vi "Brightcoveload.vi"() -> ()   [LabVIEW 2026]
uses:
  <vilib>/sklein/WebView2/Webview2 Lib/WebView2 Control Object/Paths.ctl
  <vilib>/sklein/WebView2/Webview2 Lib/WebView2 Control Object/Core Env Options.ctl
  <vilib>/sklein/WebView2 QControl/WebView2 QControl/WebView2 QControl/WebView2 QControl.lvclass/WebView2 QControl.ctl
  <userlib>/_lava_lib_tree_control.llb/CommunityTreeAPITYPEDEF - DataStore Command.ctl
  9dcc2fe5-36b0-449a-ab0d-001457c950c8.vi
  5299e24a-5130-419c-9a3c-199b24d92175.vi
  <vilib>/sklein/WebView2 QControl/WebView2 QControl/WebView2 QControl/Write Document Source.vi
  <vilib>/sklein/WebView2 QControl/WebView2 QControl/WebView2 QControl/Read Events.vi
  <vilib>/sklein/WebView2/Webview2 Lib/WebView2 Control Object/Read Events.vi
  <vilib>/sklein/WebView2/Webview2 Lib/WebView2 Control Object/Write Document Source.vi
  <vilib>/sklein/WebView2/Webview2 Lib/WebView2 Control Object/Register Events.vi
  <vilib>/JDP Science/JSONtext/Variant to JSON Text.vi
  <vilib>/JDP Science/JSONtext/LVClass Serializer/JSONtext LVClass Serializer.lvclass
  <vilib>/sklein/WebView2 QControl/WebView2 QControl/WebView2 QControl/WebView2 QControl.lvclass
  <vilib>/sklein/WebView2/Webview2 Lib/WebView2 Control Object/WebView2 Control.lvclass
  <vilib>/sklein/WebView2/Libs/Microsoft.Web.WebView2.WinForms.dll
panel:
  out "<JSON>":string
  in  "WebView2":refnum<k24>(container)
  in  "Tree":string(tree)
  in  "Tree 2":string(tree)
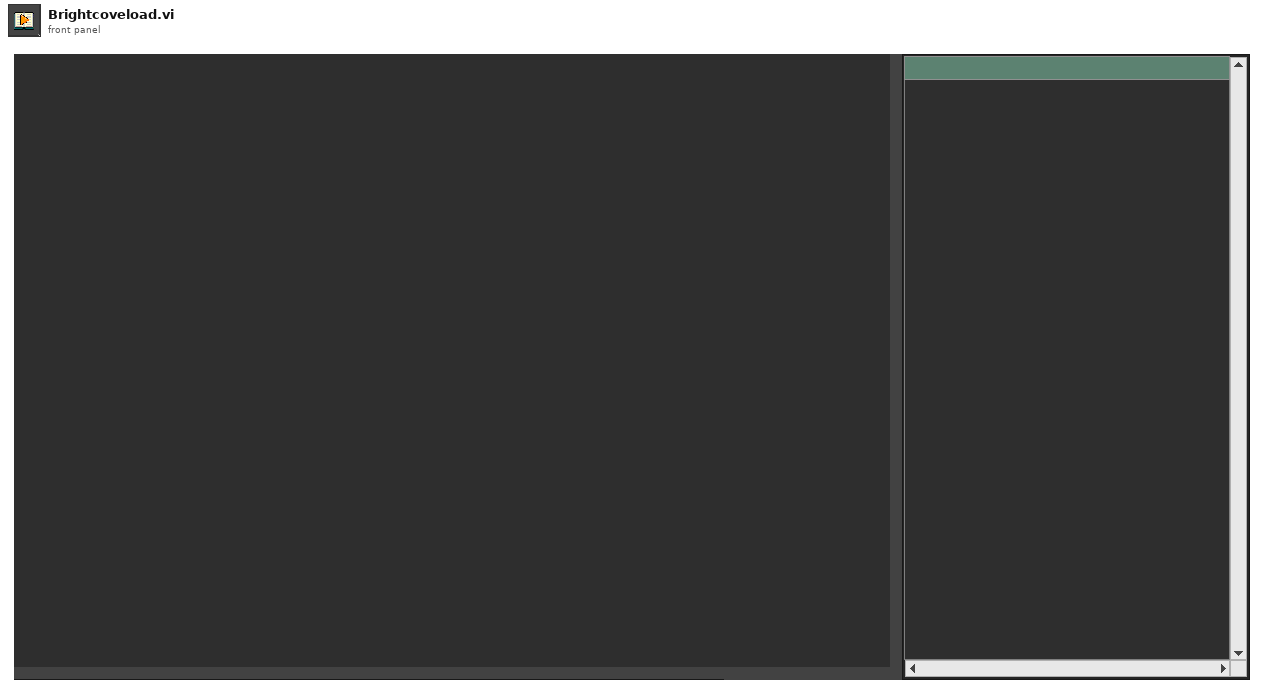
[diagram p1: front panel]
types:
  T1 = typedef "WebView2.lvlib/WebView2 Control.lvclass/Core Env Options.ctl" = cluster{"additionalBrowserArguments":string, "language":string, "targetCompatibleBrowserVersion":string, "allowSingleSignOnUsingOSPrimaryAccount":bool}
  T2 = typedef "WebView2.lvlib/WebView2 Control.lvclass/Paths.ctl" = cluster{"Webview2 Native":path, "Edge Application":path, "User Data":path}
  T3 = typedef "WebView2.lvlib/WebView2 Control.lvclass/Events.ctl" = cluster{"Navigation Complete Event":refnum<user-event>, "Source Changed Event":refnum<user-event>, "Document Title Changed Event":refnum<user-event>, "Status Bar Text Changed":refnum<user-event>, "Web Message Received":refnum<user-event>, "Window Close Requested":refnum<user-event>, "DOM Loaded":refnum<user-event>, "Navigation Started Event":refnum<user-event>}
  T4 = typedef "imagedata.ctl" = cluster{"image type":i32, "image depth":i32, "image":u8[], "mask":u8[], "colors":u32[], "Rectangle":cluster{"left":i16, "top":i16, "right":i16, "bottom":i16}}
  T5 = typedef "CommunityTreeAPITYPEDEF - DataStore Command.ctl" = enum16{"Init", "Add", "Get", "Clear Tree", "Clear All", "Modify"}
  T6 = typedef "LVRectTypeDef.ctl" = cluster{"Left":i16, "Top":i16, "Right":i16, "Bottom":i16}
  T7 = enum16{"No Scaling", "Scale All Objects", "Scale Single Object"}
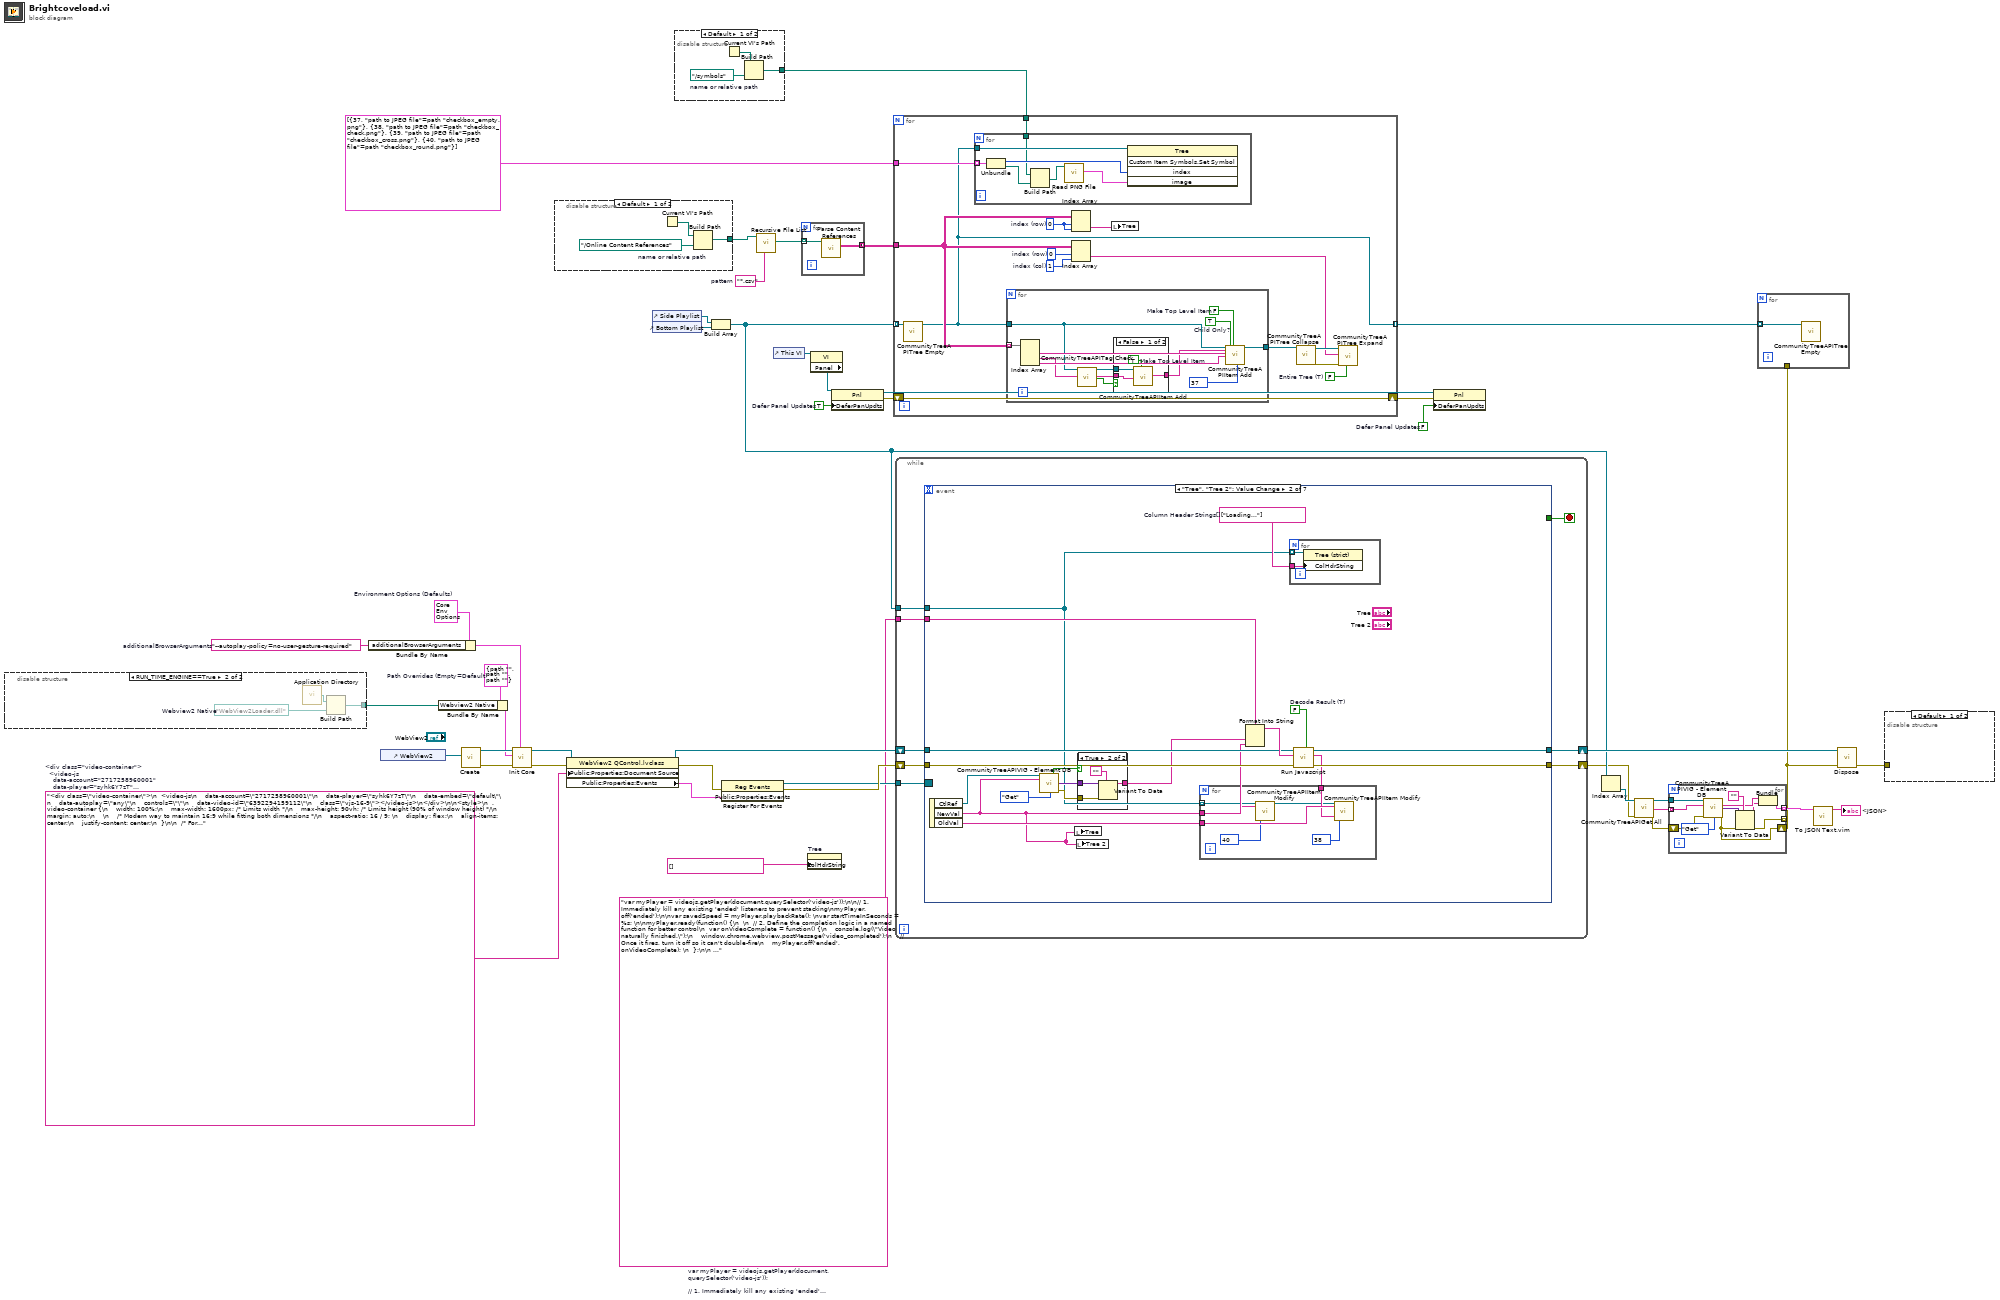
[diagram p0: block diagram]
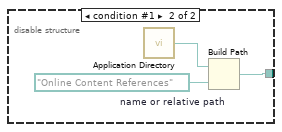
[diagram p2: hidden frame]
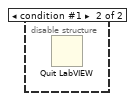
[diagram p4: hidden frame]
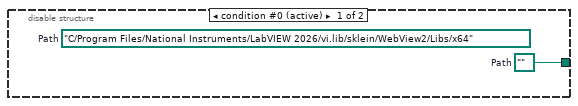
[diagram p5: hidden frame]
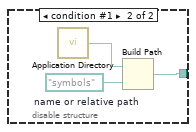
[diagram p6: hidden frame]
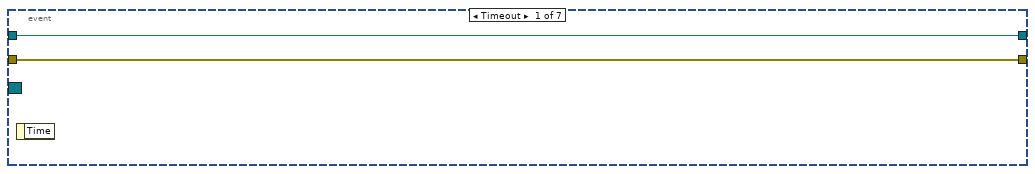
[diagram p7: hidden frame]
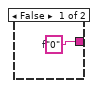
[diagram p8: hidden frame]
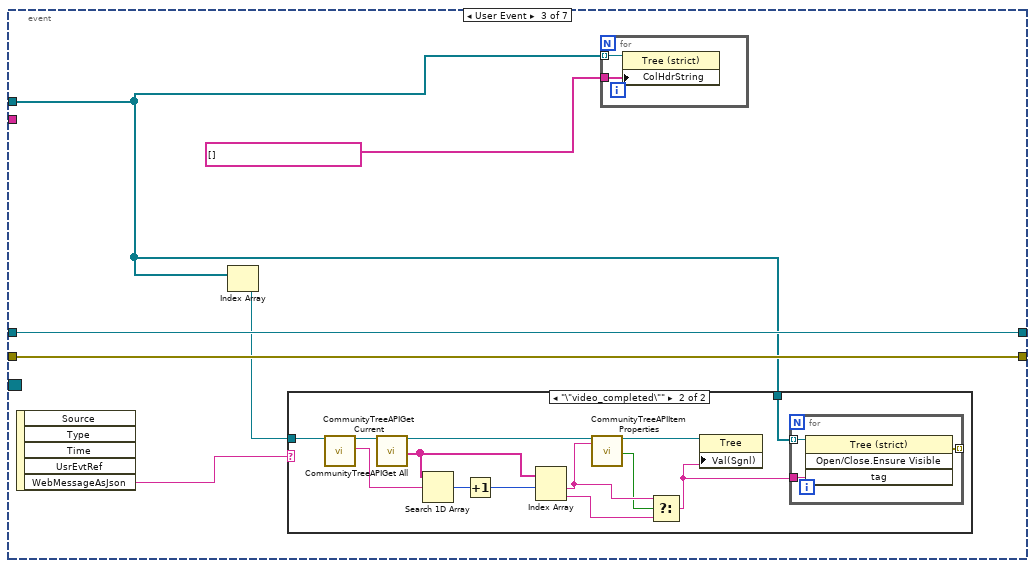
[diagram p9: hidden frame]
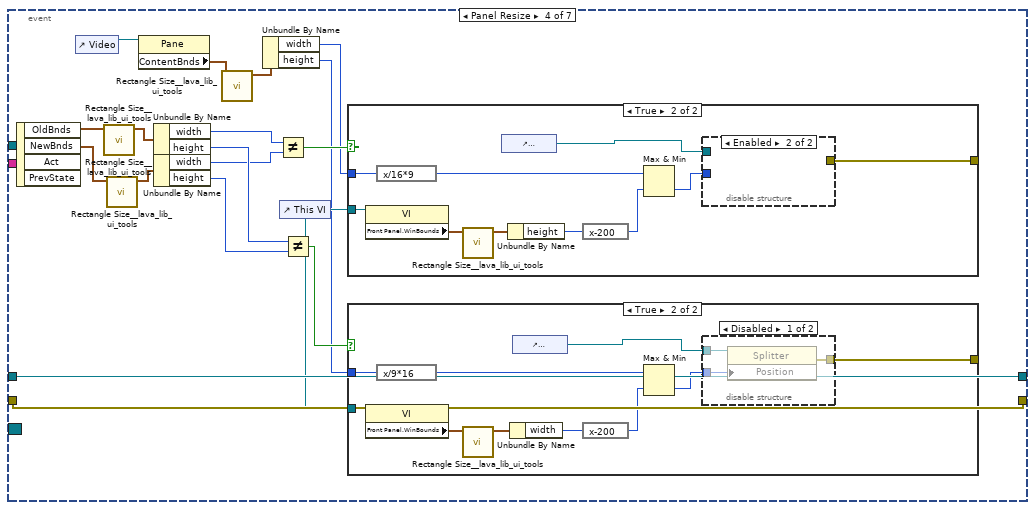
[diagram p11: hidden frame]
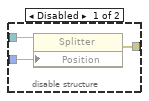
[diagram p15: hidden frame]
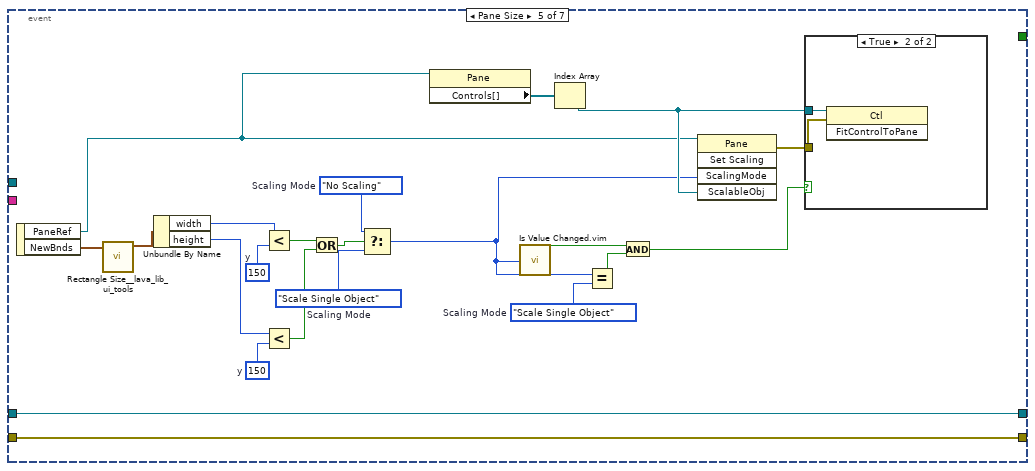
[diagram p16: hidden frame]
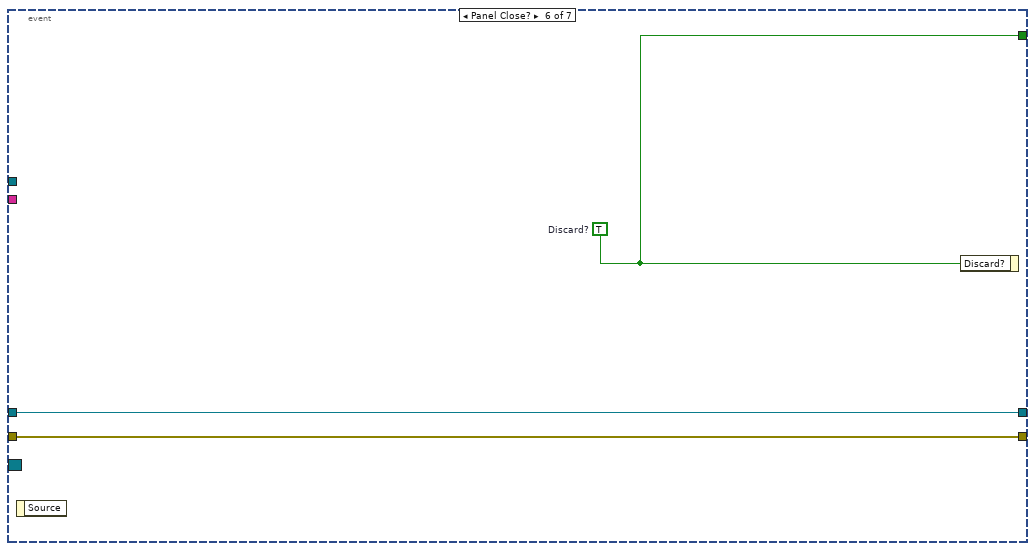
[diagram p18: hidden frame]
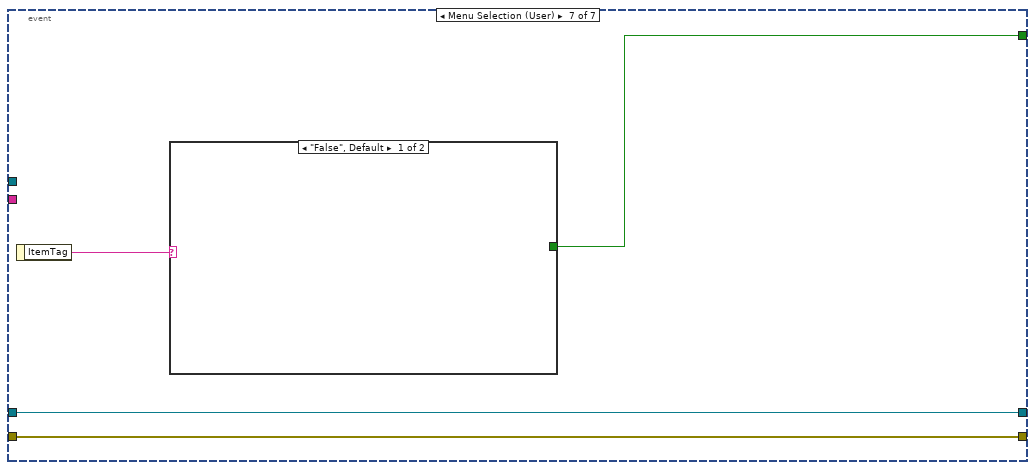
[diagram p19: hidden frame]
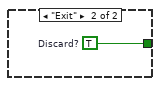
[diagram p20: hidden frame]
diagram:
  w2 = "--autoplay-policy=no-user-gesture-required"  # additionalBrowserArguments
  w4 = T1 {"additionalBrowserArguments"="--autoplay-policy=no-user-gesture-required", "language"="", "targetCompatibleBrowserVersion"="", "allowSingleSignOnUsingOSPrimaryAccount"=FALSE}  # Environment Options (Defaults)
  w16 = "*.csv"  # pattern
  w22 = FALSE  # Defer Panel Updates
  w25 = TRUE  # Defer Panel Updates
  w14 = "var myPlayer = videojs.getPlayer(document.querySelector('video-js'));\n\n// 1. Immediately kill any existing 'ended' listeners to prevent stacking\nmyPlayer.off('ended');\n\nvar savedSpeed = myPlayer.playbackRate(); \nvar startTimeInSeconds = %s; \n\nmyPlayer.ready(function() {\n  \n  // 2. Define the completion logic in a named function for better control\n  var onVideoComplete = function() {\n    console.log(\"Video naturally finished.\");\n    window.chrome.webview.postMessage('video_completed');\n    // Once it fires, turn it off so it can't double-fire\n    myPlayer.off('ended', onVideoComplete); \n  };\n\n  myPlayer.catalog.getVideo('%s', function(error, video) {\n    if (!error) {\n      // 3. Pause and reset the current source before loading the new one\n      myPlayer.pause();\n      \n      myPlayer.catalog.load(video);\n      \n      myPlayer.one('loadedmetadata', function() {\n        myPlayer.playbackRate(savedSpeed);  \n        myPlayer.currentTime(startTimeInSeconds); \n        \n        // 4. Only attach the 'ended' listener AFTER the new video is ready\n        myPlayer.on('ended', onVideoComplete);\n\n        myPlayer.play(); \n        window.chrome.webview.postMessage('abc'); \n      });\n    }\n  });\n});\nmyPlayer.currentTime();"  # var myPlayer = videojs.getPlayer(document.querySelector('video-js'));  // 1. Immediately kill any existing 'ended' listeners to prevent stacking myPlayer.off('ended');  var savedSpeed = myPlayer.playbackRate();  var startTimeInSeconds = %s;   myPlayer.ready(function() {      // 2. Define the completion logic in a named function for better control   var onVideoComplete = function() {     console.log("Video naturally finished.");     window.chrome.webview.postMessage('video_completed');     // Once it fires, turn it off so it can't double-fire     myPlayer.off('ended', onVideoComplete);    };    myPlayer.catalog.getVideo('%s', function(error, video) {     if (!error) {       // 3. Pause and reset the current source before loading the new one       myPlayer.pause();              myPlayer.catalog.load(video);              myPlayer.one('loadedmetadata', function() {         myPlayer.playbackRate(savedSpeed);           myPlayer.currentTime(startTimeInSeconds);                   // 4. Only attach the 'ended' listener AFTER the new video is ready         myPlayer.on('ended', onVideoComplete);          myPlayer.play();          window.chrome.webview.postMessage('abc');        });     }   }); }); myPlayer.currentTime();
  w34 = T2 {"Webview2 Native"=path "", "Edge Application"=path "", "User Data"=path ""}  # Path Overrides (Empty=Default)
  w40 = "<div class=\"video-container\">\n  <video-js\n    data-account=\"2717258960001\"\n    data-player=\"syhk6Y7zT\"\n    data-embed=\"default\"\n    data-autoplay=\"any\"\n    controls=\"\"\n    data-video-id=\"6392294159112\"\n    class=\"vjs-16-9\"></video-js>\n</div>\n\n<style>\n  .video-container {\n    width: 100%;\n    max-width: 1600px; /* Limits width */\n    max-height: 90vh; /* Limits height (90% of window height) */\n    margin: auto;\n    \n    /* Modern way to maintain 16:9 while fitting both dimensions */\n    aspect-ratio: 16 / 9; \n    display: flex;\n    align-items: center;\n    justify-content: center;\n  }\n\n  /* Force the video-js element to fill this constrained container */\n  .video-container video-js {\n    width: 100% !important;\n    height: 100% !important;\n    position: relative !important;\n    padding-top: 0 !important; /* Overrides the default vjs-16-9 padding */\n  }\n</style>\n<script\n  src=\"https://players.brightcove.net/2717258960001/syhk6Y7zT_default/index.min.js\">\n</script>\n"  # <div class="video-container">   <video-js     data-account="2717258960001"     data-player="syhk6Y7zT"     data-embed="default"     data-autoplay="any"     controls=""     data-video-id="6392294159112"     class="vjs-16-9"></video-js> </div>  <style>   .video-container {     width: 100%;     max-width: 1600px; /* Limits width */     max-height: 90vh; /* Limits height (90% of window height) */     margin: auto;          /* Modern way to maintain 16:9 while fitting both dimensions */     aspect-ratio: 16 / 9;      display: flex;     align-items: center;     justify-content: center;   }    /* Force the video-js element to fill this constrained container */   .video-container video-js {     width: 100% !important;     height: 100% !important;     position: relative !important;     padding-top: 0 !important; /* Overrides the default vjs-16-9 padding */   } </style> <script   src="https://players.brightcove.net/2717258960001/syhk6Y7zT_default/index.min.js"> </script>
  n1 = disable-structure shown="RUN_TIME_ENGINE==True" {
    disable-tunnel: [w47 w48] -> w27
    frame condition #0 (active) {
      (unwired) path "C:/Program Files/National Instruments/LabVIEW 2026/vi.lib/sklein/WebView2/Libs/x64"  # Path
      w47 = path ""  # Path
    }
    frame condition #1 {
      w49 = path "WebView2Loader.dll"  # Webview2 Native
      n2 = call <vilib>:"Application Directory.vi"() -> ("Application Directory"=w50:path)
      n3 = Build Path(base path=w50, name or relative path=w49) -> (appended path=w48:path)
    }
  }
  n4 = Bundle By Name(cluster=w4, "additionalBrowserArguments"=w2) -> (w3:T1)
  n5 = control-ref of="WebView2"() -> (w44:refnum<vi>)
  n6 = Bundle By Name(cluster=w34, "Webview2 Native"=w27) -> (w32:T2)
  n7 = call <vilib>:"Create.vi"("WebView2 Control Ref"=w44) -> ("error out"=w38:errorcluster, "WebView2 Control out"=w43:refnum<class "WebView2 QControl.lvclass">)  [unwired: 9 in]
  n8 = call <vilib>:"Init Core.vi"("Environment Options (Defaults)"=w3, "error in (no error)"=w38, "Path Overrides (Empty=Default)"=w32, "WebView2 Control in"=w43) -> ("error out"=w42:errorcluster, "WebView2 Control out"=w37:refnum<class "WebView2 QControl.lvclass">)  [unwired: 6 in]
  n9 = disable-structure shown="Default" {
    disable-tunnel: [w51 w54] -> w17
    frame condition #0 (active) {
      w53 = path "../Online Content References"  # name or relative path
      n10 = Current VI's Path() -> (path=w52:path)
      n11 = Build Path(base path=w52, name or relative path=w53) -> (appended path=w51:path)
    }
    frame condition #1 {
      w56 = path "Online Content References"  # name or relative path
      n12 = call <vilib>:"Application Directory.vi"() -> ("Application Directory"=w55:path)
      n13 = Build Path(base path=w55, name or relative path=w56) -> (appended path=w54:path)
    }
  }
  n14 = property class="WebView2 QControl.lvclass"(reference=w37, error in=w42, "Public:Properties:Document Source"=w40) -> (reference out=w36:refnum<class "WebView2 QControl.lvclass">, error out=w1:errorcluster, "Public:Properties:Events"=w30:T3)
  n15 = control-ref of="Side Playlist"() -> (w26:refnum<vi>)
  n16 = control-ref of="Bottom Playlist"() -> (w45:refnum<vi>)
  n17 = disable-structure shown="Default" {
    disable-tunnel: [w57 w60] -> w35
    frame condition #0 (active) {
      w59 = path "../symbols"  # name or relative path
      n18 = Current VI's Path() -> (path=w58:path)
      n19 = Build Path(base path=w58, name or relative path=w59) -> (appended path=w57:path)
    }
    frame condition #1 {
      w62 = path "symbols"  # name or relative path
      n20 = call <vilib>:"Application Directory.vi"() -> ("Application Directory"=w61:path)
      n21 = Build Path(base path=w61, name or relative path=w62) -> (appended path=w60:path)
    }
  }
  n22 = Build Array(w26, w45) -> (w13:refnum<vi>[])
  n23 = register-events(error in=w1, w30) -> (reference out=w29:refnum<event-registration>, error out=w46:errorcluster)  [unwired: 1 in]
  n24 = call <vilib>:"Recursive File List.vi"("pattern"=w16, "Folder Path"=w17) -> ("All Files in Dir"=w15:path[])  [unwired: 5 in, 4 out]
  n25 = control-ref of="This VI"() -> (w20:refnum<vi>)
  n26 = for {
    tunnel: [w64] -> w28 mode=concatenating
    tunnel: w15 -> [w63] mode=indexing
    n27 = call "Parse Content References.vi"("file path in"=w63) -> ("transposed array"=w64:string[][])  [unwired: 14 in]
  }
  n28 = property on="Tree" class="Tree (strict)"("ColHdrString"=string[] []) -> ()  [unwired: 2 in, 2 out]
  n29 = property class="VI"(reference=w20) -> ("Panel"=w19:refnum<vi>)  [unwired: 1 in, 2 out]
  n30 = property class="Pnl"(reference=w19, "DeferPanUpdts"=w25) -> (reference out=w21:refnum<vi>, error out=w24:errorcluster)  [unwired: 1 in]
  n31 = for {
    tunnel: w13 -> [w79] mode=indexing
    tunnel: cluster{i32, "path to JPEG file":path}[] [{37, "path to JPEG file"=path "checkbox_empty.png"}, {38, "path to JPEG file"=path "checkbox_check.png"}, {39, "path to JPEG file"=path "checkbox_cross.png"}, {40, "path to JPEG file"=path "checkbox_round.png"}] -> [w78]
    tunnel: w35 -> [w75]
    tunnel: w28 -> [w67]
    shift-right: [w66] -> w23
    shift-left: w24 -> [w66]
    tunnel: [w65] -> w18 mode=indexing
    w69 = 1  # index (col)
    w70 = 0  # index (row)
    w71 = FALSE  # Entire Tree (T)
    w77 = 0  # index (row)
    n32 = call <userlib>:"CommunityTreeAPITree Empty.vi"("Tree Reference In"=w79) -> ("Tree Reference Out"=w65:refnum<vi>)  [unwired: 16 in, 2 out]
    n33 = for {
      tunnel: w65 -> [w86]
      tunnel: w78 -> [w84] mode=indexing
      tunnel: w75 -> [w80]
      n34 = Unbundle(w84) -> (w83:i32, "path to JPEG file"=w82:path)
      n35 = Build Path(base path=w80, name or relative path=w82) -> (appended path=w81:path)
      n36 = call <vilib>:"Read PNG File.vi"("path to PNG file"=w81) -> ("image data"=w85:T4)  [unwired: 8 in, 2 out]
      n37 = invoke class="Tree" method="Custom Item Symbols.Set Symbol"(reference=w86, "index"=w83, "image"=w85) -> ()  [unwired: 2 in, 5 out]
    }
    n38 = for {
      tunnel: w67 -> [w99] mode=indexing
      tunnel: w65 -> [w94]
      tunnel: [w87] -> w74
      w88 = TRUE  # Child Only?
      w96 = FALSE  # Make Top Level Item
      n39 = Index Array(array=w99) -> (element #1=w97:string, element #2=w93:string, element #3=w98:string)  [unwired: 3 in]
      n40 = call <userlib>:"CommunityTreeAPITag Check.vi"("Tree Reference In"=w94, "Input Tag"=w93) -> ("Tree Reference Out"=w92:refnum<vi>, "Duplicate Tag"=w91:string, "Tag OK"=w89:bool)  [unwired: 14 in, 1 out]
      n41 = case shown="False" w89 {
        tunnel: w92 -> [w103 _]
        tunnel: w91 -> [w102 w104]
        tunnel: [w100 w104] -> w90
        frame False {
          w101 = TRUE  # Make Top Level Item
          n42 = call <userlib>:"CommunityTreeAPIItem Add.vi"("Tree Reference In"=w103, "New Text Value"=w102, "Make Top Level Item"=w101) -> ("Created Tag"=w100:string)  [unwired: 14 in, 2 out]
        }
        frame True {
        }
      }
      n43 = call <userlib>:"CommunityTreeAPIItem Add.vi"("Tree Reference In"=w94, "Parent Tag (Current)"=w90, "New Tag Value (Same as Text)"=w97, "New Text Value"=w98, "Child Only?"=w88, "Make Top Level Item"=w96, "Symbol Index (0)"=37) -> ("Tree Reference Out"=w87:refnum<vi>)  [unwired: 10 in, 2 out]
    }
    n44 = Index Array(array=w67, index (row)=w77, index (col)=w77) -> (element=w76:string)
    n45 = Index Array(array=w67, index (row)=w70, index (col)=w69) -> (element=w68:string)
    n46 = local write "Tree"(w76) -> ()
    n47 = call <userlib>:"CommunityTreeAPITree Collapse.vi"("Tree Reference In"=w74) -> ("Tree Reference Out"=w73:refnum<vi>, "error out"=w72:errorcluster)  [unwired: 17 in]
    n48 = call <userlib>:"CommunityTreeAPITree Expand.vi"("Tree Reference In"=w73, "Tag To Expand"=w68, "error in (no error)"=w72, "Entire Tree (T)"=w71) -> ()  [unwired: 14 in, 2 out]
  }
  n49 = while {
    shift-right: [w109] -> w6
    shift-left: w46 -> [w112]
    shift-right: [w110] -> w41
    shift-left: w36 -> [w111]
    tunnel: w29 -> [w107]
    tunnel: w14 -> [w106]
    tunnel: w13 -> [w105]
    stop <- w108 stop-if-true
    n50 = event shown="[1] \"Tree\", \"Tree 2\": Value Change" {
      selector: w107 -> [_ _ _ _ _ _ _]
      dyn-events: _ -> [_ _ _ _ _ _ _]
      timeout: _ -> [_ _ _ _ _ _ _]
      tunnel: w112 -> [w113 w130 w151 w187 w235 w240 w244]
      tunnel: w111 -> [w114 w128 w152 w188 w236 w241 w245]
      tunnel: [w114 w132 w152 w188 w236 w241 w245] -> w110
      tunnel: [w113 w131 w151 w187 w235 w240 w244] -> w109
      tunnel: [_ _ _ _ _ w239 w242] -> w108
      tunnel: w106 -> [_ w116 _ _ _ _ _]
      tunnel: w105 -> [_ w115 w147 _ _ _ _]
      event Timeout {
        n51 = event-data() -> ()  [unwired: 1 in, 1 out]
      }
      event "Tree", "Tree 2": Value Change {
        w118 = string[] ["Loading..."]  # Column Header Strings[]
        w127 = FALSE  # Decode Result (T)
        n52 = event-data() -> ("CtlRef"=w122:refnum<vi>, "NewVal"=w117:string, "OldVal"=w126:string)  [unwired: 1 in]
        n53 = call <userlib>:"CommunityTreeAPIVIG - Element DB.vi"("Tree Ref In"=w122, "Element Tag"=w117, "Command"=CommunityTreeAPITYPEDEF_-_DataStore_Command."Get") -> ("Found"=w120:bool, "Tree Element Data Out"=w123:variant, "error out"=w121:errorcluster)  [unwired: 7 in, 3 out]
        n54 = local write "Tree"(w117) -> ()
        n55 = local write "Tree 2"(w117) -> ()
        n56 = case shown="True" w120 {
          tunnel: w123 -> [_ w146]
          tunnel: [w142 w144] -> w119
          tunnel: w121 -> [_ w143]
          frame False {
            w142 = "0"  # f
          }
          frame True {
            n57 = Variant To Data(error in=w143, type="", Variant=w146) -> (data=w144:string)  [unwired: 1 out]
          }
        }
        n58 = Format Into String(format string=w116, w119, w117) -> (resulting string=w129:string)  [unwired: 2 in, 1 out]
        n59 = for {
          tunnel: w118 -> [w134]
          tunnel: w115 -> [w133] mode=indexing
          n60 = property on="Property Node" class="Tree (strict)"(reference=w133, "ColHdrString"=w134) -> ()  [unwired: 1 in, 2 out]
        }
        n61 = call <vilib>:"Run Javascript.vi"("Decode Result (T)"=w127, "error in (no error)"=w130, "javaScript"=w129, "WebView2 Control in"=w128) -> ("error out"=w131:errorcluster, "Result"=w125:string, "WebView2 Control out"=w132:refnum<class "WebView2 QControl.lvclass">)  [unwired: 5 in]
        n62 = for {
          tunnel: w126 -> [w141]
          tunnel: w125 -> [w140]
          tunnel: w115 -> [w139] mode=indexing
          tunnel: w117 -> [w135]
          n63 = call <userlib>:"CommunityTreeAPIItem Modify.vi"("Tree Reference In"=w139, "Tag to Modify (Current)"=w135, "Symbol(-1:No Change)"=40) -> ("Tree Reference Out"=w137:refnum<vi>)  [unwired: 14 in, 2 out]
          n64 = call <userlib>:"CommunityTreeAPIItem Modify.vi"("Tree Reference In"=w137, "Tag to Modify (Current)"=w141, "Element Data"=w140, "Symbol(-1:No Change)"=38) -> ()  [unwired: 13 in, 3 out]
        }
      }
      event User Event {
        n65 = event-data() -> ("WebMessageAsJson"=w149:string)  [unwired: 1 in, 4 out]
        n66 = Index Array(array=w147) -> (element=w148:refnum<vi>)  [unwired: 1 in]
        n67 = case shown="\"\\\"video_completed\\\"\"" w149 {
          tunnel: w148 -> [_ w164]
          tunnel: w147 -> [_ w155]
          frame Default {
          }
          frame "\"video_completed\"" {
            n68 = call <userlib>:"CommunityTreeAPIGet Current.vi"("Tree Reference In"=w164) -> ("Tree Reference Out"=w165:refnum<vi>, "Current Tag"=w163:string)  [unwired: 15 in, 2 out]
            n69 = call <userlib>:"CommunityTreeAPIGet All.vi"("Tree Reference In"=w165) -> ("Tree Reference Out"=w160:refnum<vi>, "Output Tree Items"=w154:string[])  [unwired: 15 in, 2 out]
            n70 = Search 1D Array(1D array=w154, element=w163) -> (index of element=w162:i32)  [unwired: 1 in]
            n71 = Increment(x=w162) -> (x+1=w161:i32)
            n72 = Index Array(array=w154, index #1=w161) -> (element #1=w158:string, element #2=w153:string)  [unwired: 1 in]
            n73 = call <userlib>:"CommunityTreeAPIItem Properties.vi"("Tree Reference In"=w160, "Tag (Current)"=w158) -> ("Tree Reference Out"=w159:refnum<vi>, "Child-Only?"=w157:bool)  [unwired: 10 in, 6 out]
            n74 = Select(t=w158, s=w157, f=w153) -> (s? t:f=w156:string)
            n75 = property on="Property Node" class="Tree"(reference=w159, "Val(Sgnl)"=w156) -> ()  [unwired: 1 in, 2 out]
            n76 = for {
              tunnel: w156 -> [w168]
              tunnel: w155 -> [w167] mode=indexing
              tunnel: [w166] -> _ mode=indexing
              n77 = invoke class="Tree (strict)" method="Open/Close.Ensure Visible"(reference=w167, "tag"=w168) -> (error out=w166:errorcluster)  [unwired: 2 in, 3 out]
            }
          }
        }
        n78 = for {
          tunnel: string[] [] -> [w170]
          tunnel: w147 -> [w169] mode=indexing
          n79 = property on="Property Node" class="Tree (strict)"(reference=w169, "ColHdrString"=w170) -> ()  [unwired: 1 in, 2 out]
        }
      }
      event Panel Resize {
        n80 = event-data() -> ("OldBnds"=w186:T6, "NewBnds"=w181:T6)  [unwired: 1 in, 2 out]
        n81 = control-ref of="Video"() -> (w177:refnum<vi>)
        n82 = call <vilib>:"Rectangle Size__lava_lib_ui_tools.vi"("Rectangle"=w186) -> ("Rect Size"=w185:cluster{"width":i32, "height":i32})  [unwired: 8 in, 2 out]
        n83 = call <vilib>:"Rectangle Size__lava_lib_ui_tools.vi"() -> ()  [unwired: 9 in, 3 out]
        n84 = call <vilib>:"Rectangle Size__lava_lib_ui_tools.vi"("Rectangle"=w181) -> ("Rect Size"=w184:cluster{"width":i32, "height":i32})  [unwired: 8 in, 2 out]
        n85 = property class="Pane"(reference=w177) -> ("ContentBnds"=w176:T6)  [unwired: 1 in, 2 out]
        n86 = Unbundle By Name(w185) -> ("width"=w183:i32, "height"=w180:i32)
        n87 = Unbundle By Name(w184) -> ("width"=w174:i32, "height"=w172:i32)
        n88 = call <vilib>:"Rectangle Size__lava_lib_ui_tools.vi"("Rectangle"=w176) -> ("Rect Size"=w175:cluster{"width":i32, "height":i32})  [unwired: 8 in, 2 out]
        n89 = Unbundle By Name(w175) -> ("width"=w173:i32, "height"=w171:i32)
        n90 = Not Equal?(x=w183, y=w174) -> (x != y?=w182:bool)
        n91 = control-ref of="This VI"() -> (w178:refnum<vi>)
        n92 = Not Equal?(x=w180, y=w172) -> (x != y?=w179:bool)
        n93 = case shown="True" w182 {
          tunnel: w173 -> [_ w211]
          tunnel: [_ w209] -> _
          tunnel: w178 -> [_ w207]
          frame False {
          }
          frame True {
            n94 = property class="VI"(reference=w207) -> ("Front Panel.WinBounds"=w206:T6)  [unwired: 1 in, 2 out]
            n95 = expression code="x/16*9"(w211) -> (w210:i32)
            n96 = call <vilib>:"Rectangle Size__lava_lib_ui_tools.vi"("Rectangle"=w206) -> ("Rect Size"=w205:cluster{"width":i32, "height":i32})  [unwired: 8 in, 2 out]
            n97 = control-ref of="Video<>Bottom"() -> (w202:refnum<vi>)
            n98 = Unbundle By Name(w205) -> ("height"=w204:i32)
            n99 = expression code="x-200"(w204) -> (w203:i32)
            n100 = Max & Min(x=w210, y=w203) -> (min(x,y)=w208:i32)  [unwired: 1 out]
            n101 = disable-structure shown="Enabled" {
              disable-tunnel: w202 -> [w214 _]
              disable-tunnel: [w213 _] -> w209
              disable-tunnel: w208 -> [w212 _]
              frame Disabled {
                n102 = property class="Splitter"(reference=w214, "Position"=w212) -> (error out=w213:errorcluster)  [unwired: 1 in, 1 out]
              }
              frame Enabled {
              }
            }
          }
        }
        n103 = case shown="True" w179 {
          tunnel: [_ w197] -> _
          tunnel: w178 -> [_ w195]
          tunnel: w171 -> [_ w190]
          frame False {
          }
          frame True {
            n104 = property class="VI"(reference=w195) -> ("Front Panel.WinBounds"=w194:T6)  [unwired: 1 in, 2 out]
            n105 = expression code="x/9*16"(w190) -> (w198:i32)
            n106 = call <vilib>:"Rectangle Size__lava_lib_ui_tools.vi"("Rectangle"=w194) -> ("Rect Size"=w193:cluster{"width":i32, "height":i32})  [unwired: 8 in, 2 out]
            n107 = Unbundle By Name(w193) -> ("width"=w192:i32)
            n108 = control-ref of="Video<>Side"() -> (w189:refnum<vi>)
            n109 = expression code="x-200"(w192) -> (w191:i32)
            n110 = Max & Min(x=w198, y=w191) -> (min(x,y)=w196:i32)  [unwired: 1 out]
            n111 = disable-structure shown="Disabled" {
              disable-tunnel: w189 -> [w201 _]
              disable-tunnel: [w200 _] -> w197
              disable-tunnel: w196 -> [w199 _]
              frame Disabled {
                n112 = property class="Splitter"(reference=w201, "Position"=w199) -> (error out=w200:errorcluster)  [unwired: 1 in, 1 out]
              }
              frame Enabled {
              }
            }
          }
        }
      }
      event Pane Size {
        w218 = 150  # y
        w223 = T7."Scale Single Object"  # Scaling Mode
        w229 = T7."Scale Single Object"  # Scaling Mode
        w228 = T7."No Scaling"  # Scaling Mode
        w231 = 150  # y
        n113 = event-data() -> ("PaneRef"=w219:refnum<vi>, "NewBnds"=w234:T6)  [unwired: 1 in]
        n114 = call <vilib>:"Rectangle Size__lava_lib_ui_tools.vi"("Rectangle"=w234) -> ("Rect Size"=w233:cluster{"width":i32, "height":i32})  [unwired: 8 in, 2 out]
        n115 = Unbundle By Name(w233) -> ("width"=w232:i32, "height"=w217:i32)
        n116 = Less?(x=w232, y=w231) -> (x < y?=w230:bool)
        n117 = Less?(x=w217, y=w218) -> (x < y?=w215:bool)
        n118 = Or(x=w230, y=w215) -> (x .or. y?=w216:bool)
        n119 = Select(t=w228, s=w216, f=w229) -> (s? t:f=w222:T7)
        n120 = property class="Pane"(reference=w219) -> ("Controls[]"=w227:refnum<vi>[])  [unwired: 1 in, 2 out]
        n121 = call "Is Value Changed.vim"("value"=w222) -> ("changed or first call?"=w224:bool)
        n122 = Index Array(array=w227) -> (element=w226:refnum<vi>)  [unwired: 1 in]
        n123 = Equal?(x=w222, y=w223) -> (x = y?=w221:bool)
        n124 = And(x=w224, y=w221) -> (x .and. y?=w220:bool)
        n125 = invoke class="Pane" method="Set Scaling"(reference=w219, "ScalingMode"=w222, "ScalableObj"=w226) -> (error out=w225:errorcluster)  [unwired: 2 in, 4 out]
        n126 = case shown="True" w220 {
          tunnel: w226 -> [_ w238]
          tunnel: w225 -> [_ w237]
          frame False {
          }
          frame True {
            n127 = invoke class="Ctl" method="FitControlToPane"(reference=w238, error in=w237) -> ()  [unwired: 1 in, 3 out]
          }
        }
      }
      event Panel Close? {
        w239 = TRUE  # Discard?
        n128 = event-data() -> ()  [unwired: 1 in, 1 out]
        n129 = event-data("Discard?"=w239) -> ()  [unwired: 1 in, 1 out]
      }
      event Menu Selection (User) {
        n130 = event-data() -> ("ItemTag"=w243:string)  [unwired: 1 in]
        n131 = case shown="\"False\", Default" w243 {
          tunnel: [_ w246] -> w242
          frame "False", Default {
          }
          frame "Exit" {
            w246 = TRUE  # Discard?
          }
        }
      }
    }
  }
  n132 = property class="Pnl"(reference=w21, error in=w23, "DeferPanUpdts"=w22) -> ()  [unwired: 2 out]
  n133 = Index Array(array=w13) -> (element=w12:refnum<vi>)  [unwired: 1 in]
  n134 = call <userlib>:"CommunityTreeAPIGet All.vi"("Tree Reference In"=w12, "error in (no error)"=w6) -> ("Tree Reference Out"=w11:refnum<vi>, "Output Tree Items"=w10:string[], "error out"=w7:errorcluster)  [unwired: 14 in, 1 out]
  n135 = for {
    tunnel: w11 -> [w256]
    tunnel: w10 -> [w255] mode=indexing
    tunnel: [w250] -> w9 mode=indexing
    shift-right: [w248] -> w5
    shift-left: w7 -> [w249]
    tunnel: [w247] -> _ mode=indexing
    n136 = call <userlib>:"CommunityTreeAPIVIG - Element DB.vi"("Tree Ref In"=w256, "Element Tag"=w255, "error in (no error)"=w249, "Command"=CommunityTreeAPITYPEDEF_-_DataStore_Command."Get") -> ("Element Tag Out"=w252:string, "Tree Element Data Out"=w254:variant, "error out"=w248:errorcluster)  [unwired: 6 in, 3 out]
    n137 = Variant To Data(error in=w248, type="", Variant=w254) -> (data=w251:string, error out=w247:errorcluster)
    n138 = Bundle("Element Tag Out"=w252, w251) -> (w250:cluster{"Element Tag Out":string, string})  [unwired: 1 in]
  }
  n139 = for {
    tunnel: w18 -> [w258] mode=indexing
    tunnel: w5 -> [_]
    n140 = call <userlib>:"CommunityTreeAPITree Empty.vi"("Tree Reference In"=w258) -> ()  [unwired: 16 in, 3 out]
  }
  n141 = call "To JSON Text.vim"("Anything"=w9) -> ("<JSON>"=→"<JSON>":string)  [unwired: 9 in, 1 out]
  n142 = call <vilib>:"Dispose.vi"("error in (no error)"=w5, "WebView2 Control in"=w41) -> ("error out"=w33:errorcluster)  [unwired: 9 in]
  n143 = disable-structure shown="Default" {
    disable-tunnel: w33 -> [_ _]
    frame condition #0 (active) {
    }
    frame condition #1 {
      n144 = Quit LabVIEW() -> ()  [unwired: 1 in]
    }
  }
